vi "Apply special move.vi"(8 "error in (no error)":errorcluster, 10 "Position in":refnum<class "Position.lvclass">, 11 "Castling in":refnum<class "Castling.lvclass">) -> (0 "error out":errorcluster, 2 "Position out":refnum<class "Position.lvclass">, 3 "Castling out":refnum<class "Castling.lvclass">)   [LabVIEW 2016, in "Chesslib.lvlib" / "Castling.lvclass"]
uses:
  Castling.lvclass
  Position/Position.lvclass
  Castling.lvclass/Castling.ctl
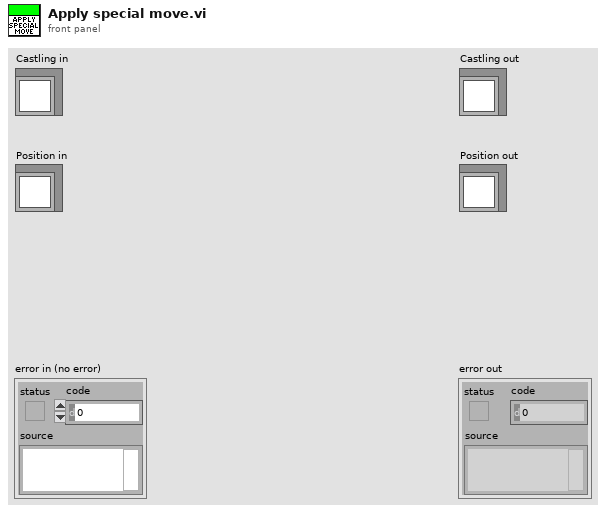
[diagram p1: front panel]
types:
  T1 = typedef "Chesslib.lvlib/Square.ctl" = cluster{"File":T2, "Rank":T3}
  T2 = typedef "Chesslib.lvlib/File.ctl" = enum8{"a", "b", "c", "d", "e", "f", "g", "h"}
  T3 = typedef "Chesslib.lvlib/Rank.ctl" = enum8{"1", "2", "3", "4", "5", "6", "7", "8"}
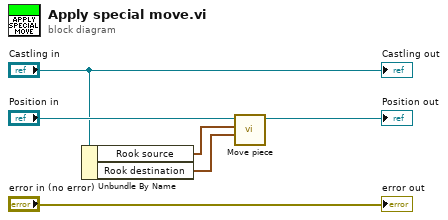
[diagram p0: block diagram]
diagram:
  n1 = Unbundle By Name("Castling in") -> ("Rook source"=w2:T1, "Rook destination"=w1:T1)
  n2 = call "Move piece.vi"("Destination"=w1, "Source"=w2, "Position in"="Position in") -> ("Position out"=→"Position out":refnum<class "Position.lvclass">)  [unwired: 5 in, 3 out]
  "error out" <- "error in (no error)"
  "Castling out" <- "Castling in"
